vi "H5Tget_fields.vi"(8 "error in (no error)":errorcluster, 11 "HDF5 Ref":T1) -> (0 "error out":errorcluster, 1 "matissa size":u32, 2 "mantissa pos":u32, 3 "HDF5 Ref out":T1, 4 "exponent pos":u32, 5 "sign pos":u32, 6 "exponent size":u32)   [LabVIEW 2017]
doc: "Retrieves floating point datatype bit field information."
uses:
  <vilib>/UPVI/lvhdf5/library.llb/HDF5 Ref.ctl
  <vilib>/UPVI/lvhdf5/hdf5.dll
panel:
  # "LVHDF5 Toolkit\nCopyright (c) 2005-2013 by Jason D. Sommerville\nCopyright (c) 2014 by UPVI, LLC.\n\nThis use and distribution of this file is governed by the terms found in \nLICENSE.txt distributed with this toolkit and installed at\n <user.lib>\\_lvhdf5\\LICENSE.txt"
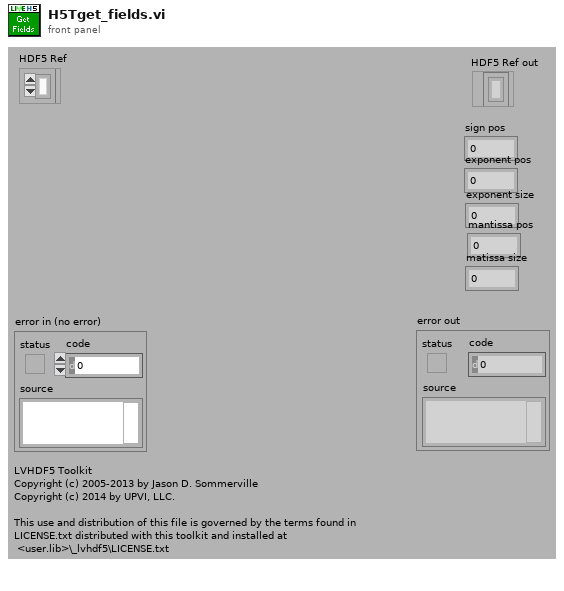
[diagram p1: front panel]
types:
  T1 = typedef "HDF5 Ref.ctl" = refnum<k1>
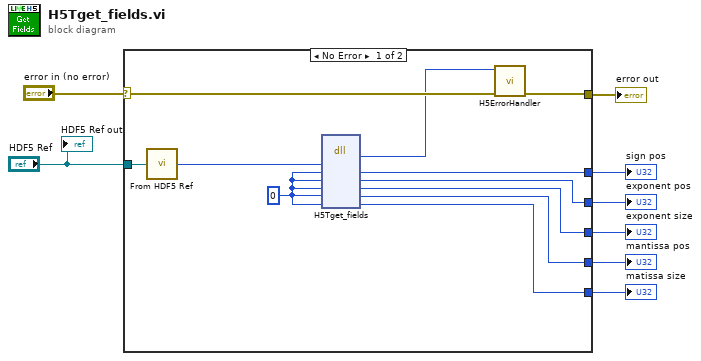
[diagram p0: block diagram]
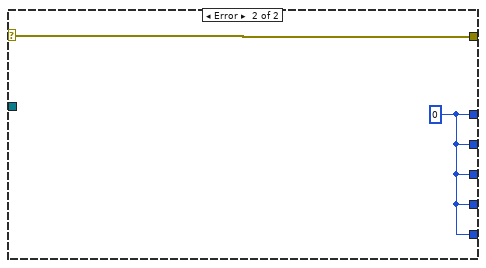
[diagram p2: hidden frame]
diagram:
  n1 = case shown="No Error" "error in (no error)" {
    selector: "error in (no error)" -> [w19 w21]
    tunnel: [w18 w21] -> w7
    tunnel: "HDF5 Ref" -> [w16 _]
    tunnel: [w13 w20] -> w5
    tunnel: [w12 w20] -> w4
    tunnel: [w11 w20] -> w3
    tunnel: [w10 w20] -> w2
    tunnel: [w9 w20] -> w1
    frame No Error {
      w14 = u64 0
      n2 = call <vilib>:"From HDF5 Ref.vi"("HDF5 Ref"=w16) -> ("I32"=w15:i32)
      n3 = dll-call lib="C:/Program Files/National Instruments/LabVIEW 2017/vi.lib/UPVI/lvhdf5/hdf5.dll" fn="H5Tget_fields"("type_id"=w15, "spos"=w14, "epos"=w14, "esize"=w14, "mpos"=w14, "msize"=w14) -> ("return type"=w17:i32, "spos"=w13:u64, "epos"=w12:u64, "esize"=w11:u64, "mpos"=w10:u64, "msize"=w9:u64)  [unwired: 4 in, 2 out]
      n4 = call <vilib>:"H5ErrorHandler.vi"("error in (no error)"=w19, "herr_t"=w17) -> ("error out"=w18:errorcluster)  [unwired: 3 in, 4 out]
    }
    frame Error {
      w20 = u32 0 ("spos")
    }
  }
  "error out" <- w7
  "sign pos" <- w5
  "exponent pos" <- w4
  "exponent size" <- w3
  "mantissa pos" <- w2
  "matissa size" <- w1
  "HDF5 Ref out" <- "HDF5 Ref"
